vi "Gui.Translate.Choose.vi"(8 "error in":errorcluster) -> (0 "error out":errorcluster, 2 "changed":bool)   [LabVIEW 2019, in "TemplateModule.lvlib"]
uses:
  TemplateModule.lvlib
  Tools/TMOS config/TMOS.Config.Action.ctl
  Tools/TMOS/Path/TMOS.Path.Type.ctl
  <vilib>/regexp/Match Regular Expression.xnode
  Tools/Translator/Translator.Language.ctl
  Tools/Tools.lvlib
  Gui.Translate.Choose.State.vi
panel:
  out "TMOS settings":cluster{"Language":string}={"Language"="English"}
  in  "OK Button":bool
  in  "Next Language Button":bool
  in  "Previous Language Button":bool
  out "languages":T1[](array[typedef])
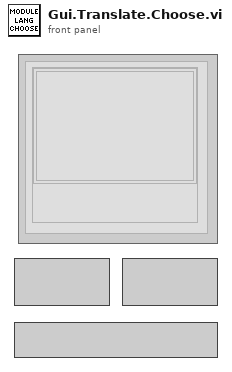
[diagram p1: front panel]
types:
  T1 = typedef "Tools.lvlib/Translator.Language.ctl" = cluster{"flag":picture, "name":string}
  T2 = typedef "TemplateModule.lvlib/Gui.Translate.Choose.State.vi" = enum16{"init", "idle", "quit"}
  T3 = typedef "TMOS.Config.Action.ctl" = enum16{"init", "update", "get", "set"}
  T4 = typedef "TMOS.Path.Type.ctl" = enum16{"TMOS Configuration file", "Resources directory", "Root directory", "Settings directory", "Verification file", "Users file", "Logs directory", "Drivers directory"}
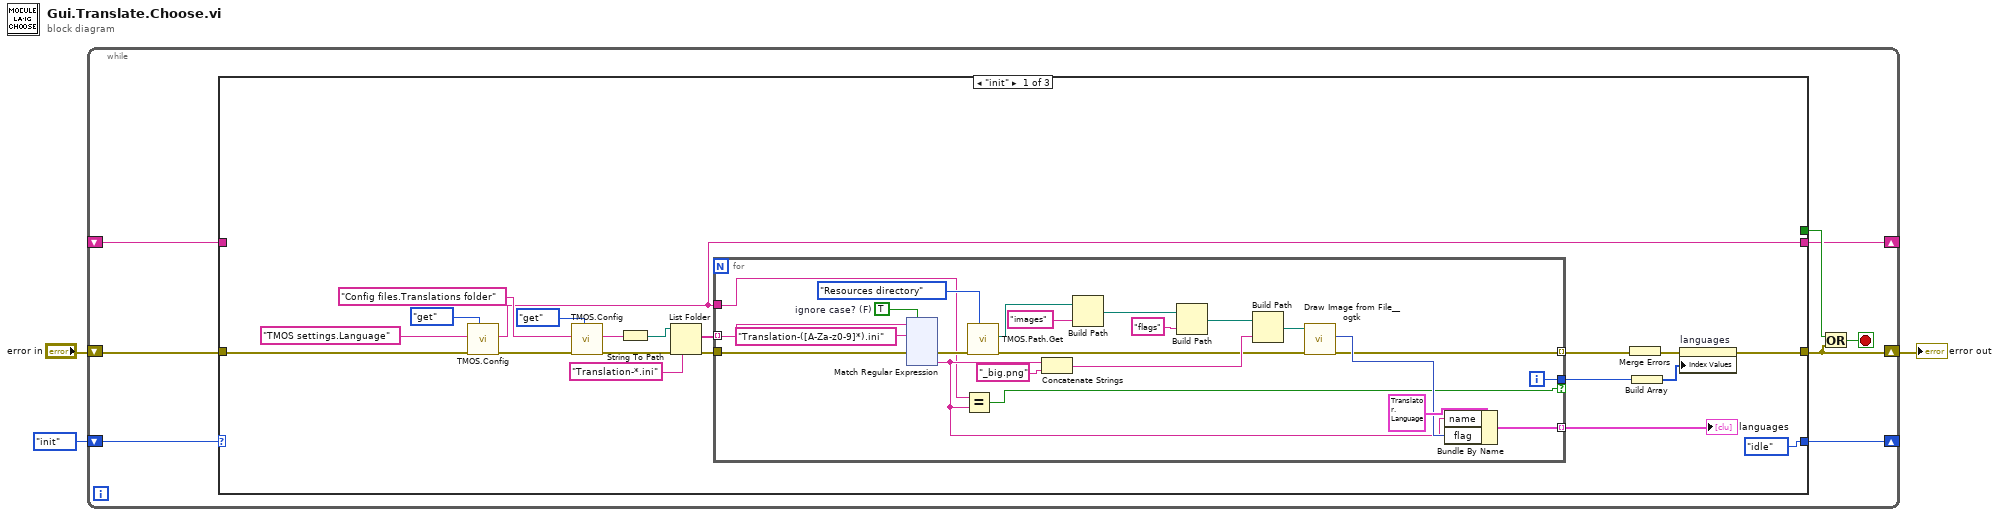
[diagram p0: block diagram]
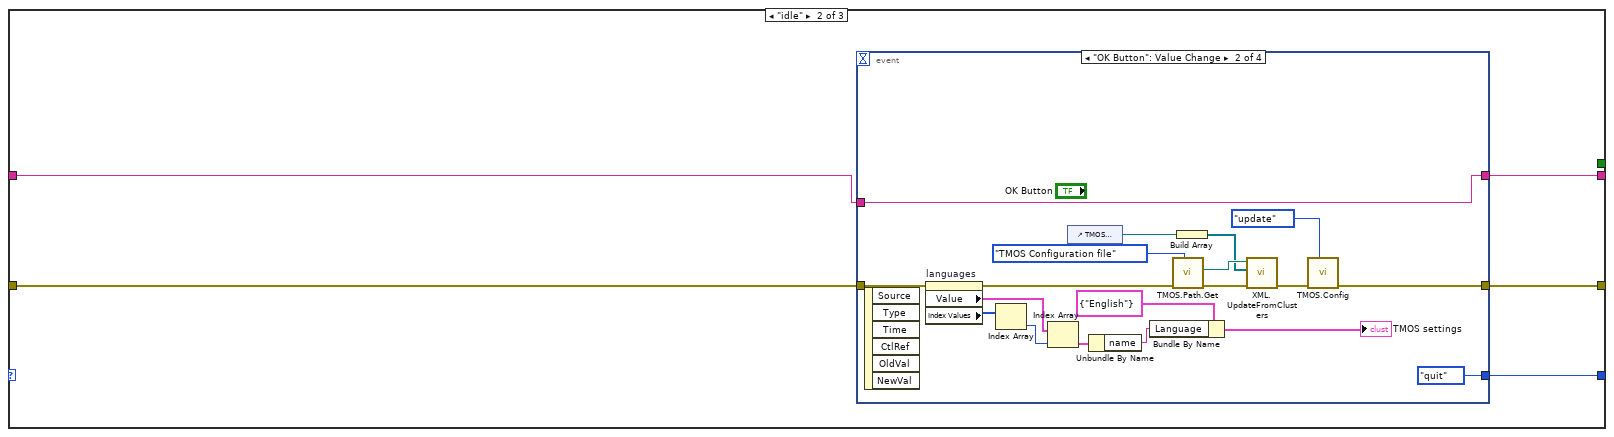
[diagram p2: hidden frame]
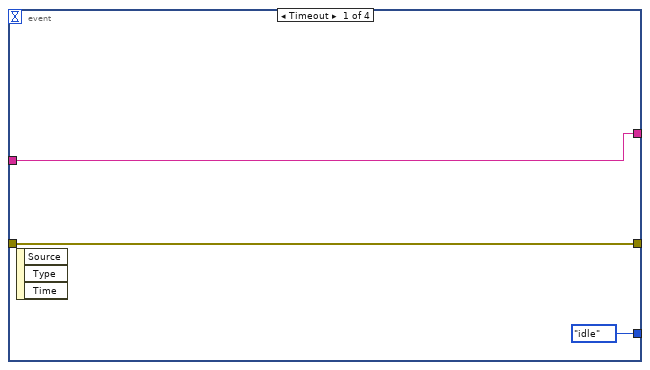
[diagram p3: hidden frame]
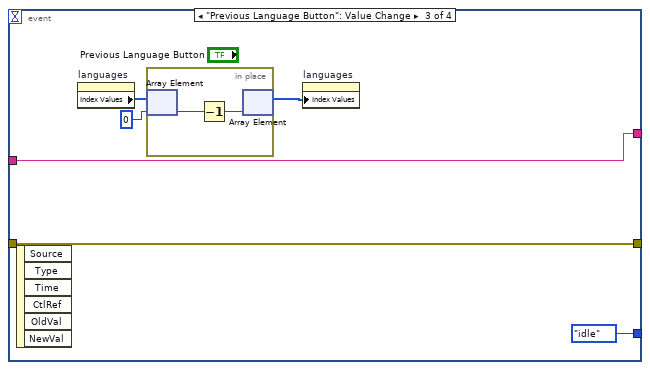
[diagram p4: hidden frame]
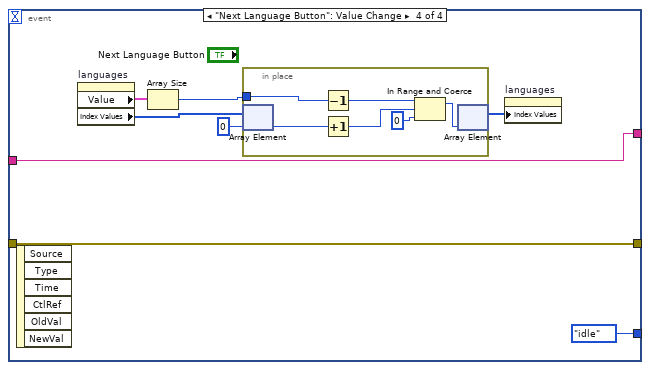
[diagram p5: hidden frame]
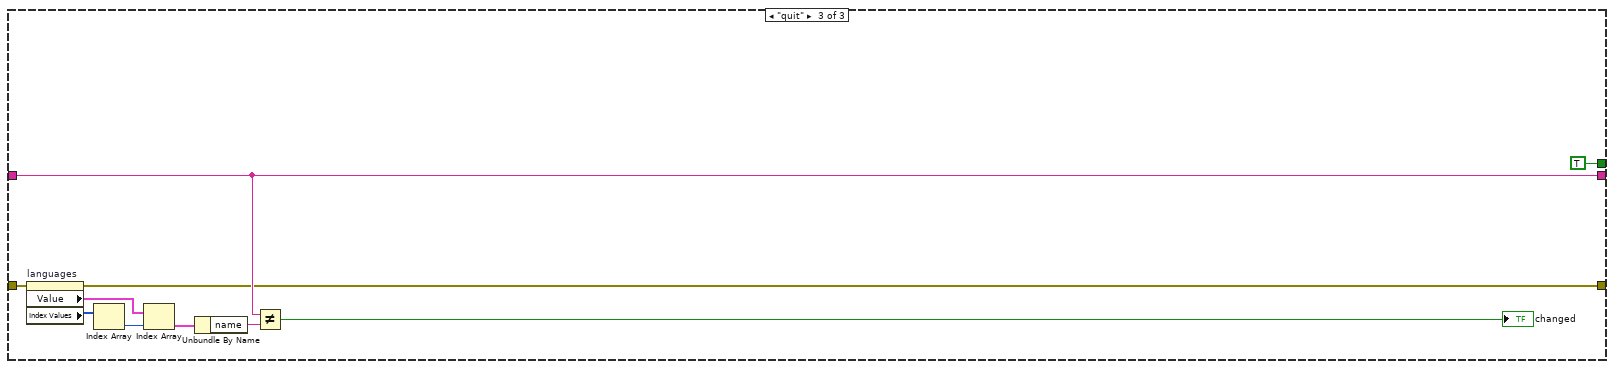
[diagram p6: hidden frame]
diagram:
  n1 = while {
    shift-right: [w9] -> _
    shift-left: Gui.Translate.Choose.State.vi."init" -> [w11]
    shift-right: [w6] -> w1
    shift-left: "error in" -> [w10]
    shift-right: [w5] -> _
    shift-left: _ -> [w4]
    stop <- w7 stop-if-true
    n2 = case shown="\"init\"" w11 {
      tunnel: [w13 w175 w220] -> w6
      tunnel: w10 -> [w18 w174 w221]
      tunnel: [Gui.Translate.Choose.State.vi."idle" w173 _] -> w9
      tunnel: [_ _ TRUE] -> w8
      tunnel: [w12 w172 w223] -> w5
      tunnel: w4 -> [_ w171 w223]
      frame "init" {
        n3 = call "TMOS.Config.vi"("action"=TMOS.Config.Action."get", "error in"=w18, "name"="TMOS settings.Language" ("~Language in use")) -> ("error out"=w17:errorcluster, "read value"=w12:string)  [unwired: 6 in, 1 out]
        n4 = call "TMOS.Config.vi"("action"=TMOS.Config.Action."get", "error in"=w17, "name"="Config files.Translations folder" ("~Language in use")) -> ("error out"=w26:errorcluster, "read value"=w22:string)  [unwired: 6 in, 1 out]
        n5 = String To Path(string=w22) -> (path=w25:path)
        n6 = List Folder(path=w25, pattern="Translation-*.ini", error in=w26) -> (filenames=w28:string[], error out=w29:errorcluster)  [unwired: 1 in, 2 out]
        n7 = for {
          tunnel: w28 -> [w54] mode=indexing
          tunnel: w29 -> [w52]
          tunnel: [w37] -> w30 mode=indexing
          tunnel: [w36] -> w31 mode=indexing
          tunnel: w12 -> [w34]
          tunnel: [w33] -> w16 if=w32
          i -> [w33]
          w51 = TRUE  # ignore case? (F)
          n8 = xnode "Match Regular Expression"("input string"=w54, "regular expression"="Translation-([A-Za-z0-9]*).ini", "error in"=w52, "ignore case? (F)"=w51) -> ("error out"=w42:errorcluster, "submatch 1"=w35:string)  [unwired: 2 in, 4 out]
          n9 = Equal?(x=w34, y=w35) -> (x = y?=w32:bool)
          n10 = call "TMOS.Path.Get.vi"("type"=TMOS.Path.Type."Resources directory", "error in"=w42) -> ("error out"=w38:errorcluster, "path"=w49:path)  [unwired: 7 in, 1 out]
          n11 = Concatenate Strings(w35, "_big.png" ("string")) -> (w44:string)
          n12 = Build Path(base path=w49, name or relative path="images") -> (appended path=w47:path)
          n13 = Build Path(base path=w47, name or relative path="flags") -> (appended path=w45:path)
          n14 = Build Path(base path=w45, name or relative path=w44) -> (appended path=w40:path)
          n15 = call <userlib>:"Draw Image from File__ogtk.vi"("error in (no error)"=w38, "path to image file"=w40) -> ("error out"=w37:errorcluster, "new picture"=w39:picture)  [unwired: 6 in, 2 out]
          n16 = Bundle By Name(cluster=T1 {"flag"=bytes[0], "name"=""} ("language"), "name"=w35, "flag"=w39) -> (w36:T1)
        }
        "languages" <- w31
        n17 = Merge Errors(w30) -> (w14:errorcluster)
        n18 = Build Array(w16) -> (w15:i32[])
        n19 = property on="languages" class="Arr (strict)"(error in=w14, "Index Values"=w15) -> (error out=w13:errorcluster)  [unwired: 1 in, 1 out]
      }
      frame "idle" {
        n20 = event shown="[1] \"OK Button\": Value Change" {
          selector: _ -> [_ _ _ _]
          dyn-events: _ -> [_ _ _ _]
          timeout: _ -> [_ _ _ _]
          tunnel: [w177 w193 w201 w211] -> w175
          tunnel: w174 -> [w177 w180 w201 w211]
          tunnel: [Gui.Translate.Choose.State.vi."idle" Gui.Translate.Choose.State.vi."quit" Gui.Translate.Choose.State.vi."idle" Gui.Translate.Choose.State.vi."idle"] -> w173
          tunnel: [w176 w181 w198 w206] -> w172
          tunnel: w171 -> [w176 w181 w198 w206]
          event Timeout {
            n21 = event-data() -> ()  [unwired: 1 in, 3 out]
          }
          event "OK Button": Value Change {
            n22 = event-data() -> ()  [unwired: 1 in, 6 out]
            n23 = property on="languages" class="Arr (strict)"(error in=w180) -> (error out=w179:errorcluster, "Value"=w197:T1[], "Index Values"=w196:u32[])  [unwired: 1 in, 1 out]
            n24 = Index Array(array=w196) -> (element=w195:u32)  [unwired: 1 in]
            n25 = Index Array(array=w197, index=w195) -> (element=w194:T1)
            n26 = control-ref of="TMOS settings"() -> (w187:refnum<vi>)
            n27 = Unbundle By Name(w194) -> ("name"=w183:string)
            n28 = Bundle By Name(cluster=cluster{"Language":string} {"Language"="English"} ("TMOS settings"), "Language"=w183) -> (→"TMOS settings":cluster{"Language":string})
            n29 = call "TMOS.Path.Get.vi"("type"=TMOS.Path.Type."TMOS Configuration file", "error in"=w179) -> ("error out"=w189:errorcluster, "path"=w188:path)  [unwired: 7 in, 1 out]
            n30 = Build Array(w187) -> (w186:refnum<vi>[])
            n31 = call "XML.UpdateFromClusters.vi"("error in"=w189, "Clusters refs"=w186, "XML file path"=w188) -> ("error out"=w185:errorcluster)  [unwired: 8 in]
            n32 = call "TMOS.Config.vi"("action"=TMOS.Config.Action."update", "error in"=w185) -> ("error out"=w193:errorcluster)  [unwired: 7 in, 2 out]
          }
          event "Previous Language Button": Value Change {
            n33 = event-data() -> ()  [unwired: 1 in, 6 out]
            n34 = property on="languages" class="Arr (strict)"() -> ("Index Values"=w203:u32[])  [unwired: 2 in, 2 out]
            n35 = in-place {
              n36 = in-place-array #1(w203, 0) -> (w205:u32)
              n37 = Decrement(x=w205) -> (x-1=w204:u32)
              n38 = in-place-array #1(w204) -> (w202:u32[])  [unwired: 1 out]
            }
            n39 = property on="languages" class="Arr (strict)"("Index Values"=w202) -> ()  [unwired: 2 in, 2 out]
          }
          event "Next Language Button": Value Change {
            n40 = event-data() -> ()  [unwired: 1 in, 6 out]
            n41 = property on="languages" class="Arr (strict)"() -> ("Value"=w207:T1[], "Index Values"=w213:u32[])  [unwired: 2 in, 2 out]
            n42 = Array Size(array=w207) -> (size(s)=w208:i32)
            n43 = in-place {
              in-place-border: w208 -> [w217]
              n44 = in-place-array #2(w213, 0) -> (w215:u32)
              n45 = Decrement(x=w217) -> (x-1=w216:i32)
              n46 = Increment(x=w215) -> (x+1=w214:u32)
              n47 = In Range and Coerce(upper limit=w216, x=w214, lower limit=u32 0) -> (coerced(x)=w218:u32)  [unwired: 1 out]
              n48 = in-place-array #2(w218) -> (w212:u32[])  [unwired: 1 out]
            }
            n49 = property on="languages" class="Arr (strict)"("Index Values"=w212) -> ()  [unwired: 2 in, 2 out]
          }
        }
      }
      frame "quit" {
        n50 = property on="languages" class="Arr (strict)"(error in=w221) -> (error out=w220:errorcluster, "Value"=w228:T1[], "Index Values"=w227:u32[])  [unwired: 1 in, 1 out]
        n51 = Index Array(array=w227) -> (element=w225:u32)  [unwired: 1 in]
        n52 = Index Array(array=w228, index=w225) -> (element=w226:T1)
        n53 = Unbundle By Name(w226) -> ("name"=w224:string)
        n54 = Not Equal?(x=w223, y=w224) -> (x != y?=→"changed":bool)
      }
    }
    n55 = Or(x=w8, y=w6) -> (x .or. y?=w7:bool)
  }
  "error out" <- w1
